vi "Driver - DTACQ - Send Synchronous Message.vi"(8 "error in":errorcluster, 10 "Message to Send":string, 11 "DTACQ Connection Data In":T1={"Description"="", "Address"="", "Port"=0, "timeout (ms)"=5000, "Termination Character"="\n", "TCP Connection Reference"=refnum, "Open Connection"=FALSE}) -> (0 "error out":errorcluster, 1 "Timed Out":bool=TRUE, 2 "Read String":string, 3 "DTACQ Connection Data Out":T1={"Description"="", "Address"="", "Port"=0, "timeout (ms)"=5000, "Termination Character"="\n", "TCP Connection Reference"=refnum, "Open Connection"=FALSE})   [LabVIEW 2017, in "Communications Library.lvlib"]
doc: "Writes a string to a DTACQ device using TCP and reads the response.\n\nOpens the TCP connection, if it is not already open."
uses:
  Communications Library.lvlib
  Typedefs/DTACQ Connection Data--Cluster.ctl
  <vilib>/Utility/error.llb/Clear Errors.vi
  Debug - Lower Level - Logging Tool.vi
  Error 5102 - DTACQ unit replied with an error--const.vi
  <vilib>/Utility/error.llb/Error Cluster From Error Code.vi
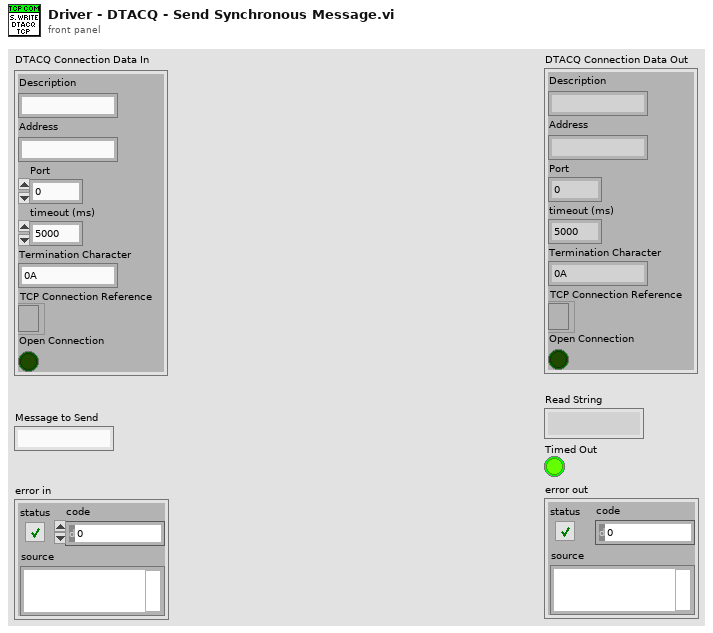
[diagram p1: front panel]
types:
  T1 = typedef "Communications Library.lvlib/DTACQ Connection Data--Cluster.ctl" = cluster{"Description":string, "Address":string, "Port":u16, "timeout (ms)":i32, "Termination Character":string, "TCP Connection Reference":refnum<k5>, "Open Connection":bool}
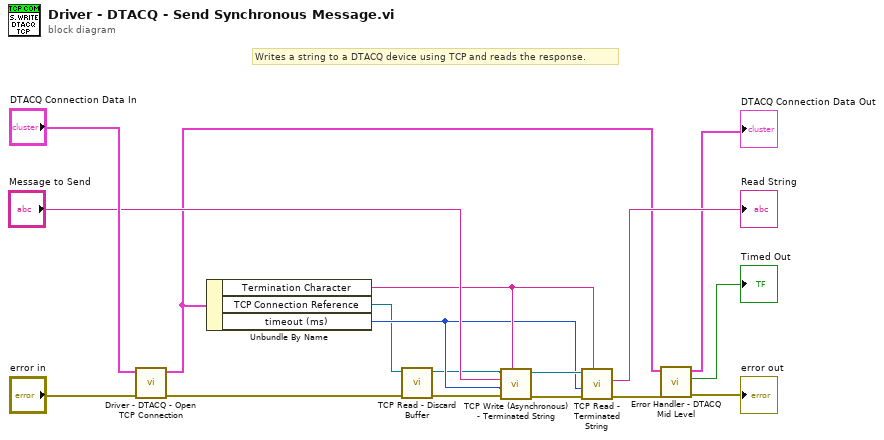
[diagram p0: block diagram]
diagram:
  # "Writes a string to a DTACQ device using TCP and reads the response."
  n1 = call "Driver - DTACQ - Open TCP Connection.vi"("error in"="error in", "DTACQ Connection Data In"="DTACQ Connection Data In") -> ("error out"=w15:errorcluster, "DTACQ Connection Data Out"=w4:T1)  [unwired: 8 in]
  n2 = Unbundle By Name(w4) -> ("Termination Character"=w12:string, "TCP Connection Reference"=w2:refnum<k5>, "timeout (ms)"=w9:i32)
  n3 = call "TCP Read - Discard Buffer.vi"("error in"=w15, "TCP Network Connection in"=w2) -> ("error out"=w14:errorcluster, "TCP Network Connection out"=w1:refnum<k5>)  [unwired: 7 in, 1 out]
  n4 = call "TCP Write (Asynchronous) - Terminated String.vi"("Termination Character"=w12, "error in"=w14, "Timeout ms (default 50ms)"=w9, "Message to Send"="Message to Send", "TCP Network Connection in"=w1) -> ("error out"=w11:errorcluster, "TCP Network Connection out"=w10:refnum<k5>)  [unwired: 5 in]
  n5 = call "TCP Read - Terminated String.vi"("Termination Character"=w12, "error in"=w11, "Timeout ms (default 50ms)"=w9, "TCP Network Connection in"=w10) -> ("error out"=w7:errorcluster, "Read String"=→"Read String":string)  [unwired: 5 in, 1 out]
  n6 = call "Error Handler - DTACQ Mid Level.vi"("error in"=w7, "DTACQ Connection Data In"=w4) -> ("error out"=→"error out":errorcluster, "Timed Out"=→"Timed Out":bool, "DTACQ Connection Data Out"=→"DTACQ Connection Data Out":T1)  [unwired: 7 in]
